vi "Begin.vi"(8 "error in":errorcluster) -> (0 "error out":errorcluster)   [LabVIEW 2020]
doc: "Called before other user functions, this VI is expected to open initial I/O refnums, load in file data, and do all program initialization. Notice that the <B>error out</B> terminal is simply used for data flow. Wiring it to other structures or subVIs ensures that this VI runs first."
uses:
  <vilib>/Rock Robotics/WPI/DriverStation/WPI_DriverStationRobotMode2.ctl
  Robot Global Data.vi
  <vilib>/Rock Robotics/Network Tables/NT Write String Array.vi
panel:
  in  "Drive Can Id":T1={"Front Left Drive CAN"=2, "Front Right Drive CAN"=3, "Back Left Drive CAN"=8, "Back Right Drive CAN"=5}
  in  "Steer Can Id":T2={"Front Left  Steer CAN"=6, "Front Right Steer CAN"=7, "Back Left Steer CAN"=9, "Back Right Steer CAN"=4}
  in  "Wheel Base Width":dbl=24.0
  in  "Wheel Base Length":dbl=24.0
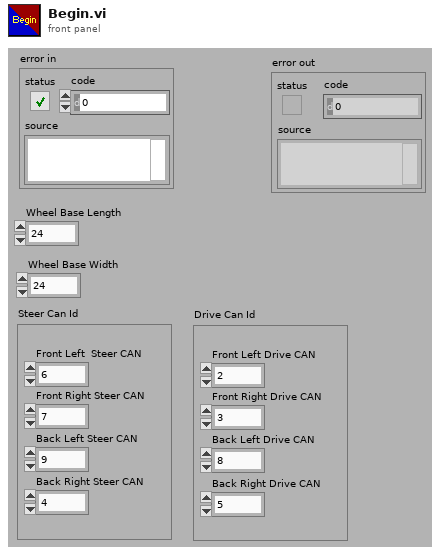
[diagram p1: front panel]
types:
  T1 = cluster{"Front Left Drive CAN":u8, "Front Right Drive CAN":u8, "Back Left Drive CAN":u8, "Back Right Drive CAN":u8}
  T2 = cluster{"Front Left  Steer CAN":u8, "Front Right Steer CAN":u8, "Back Left Steer CAN":u8, "Back Right Steer CAN":u8}
  T3 = typedef "WPI_DriverStationRobotMode2.ctl" = enum16{"Autonomous Disabled", "Autonomous Enabled", "Teleop Disabled", "Teleop Enabled", "Disconnected", "Finish", "Test Disabled", "Test Enabled", "Emergency Stopped"}
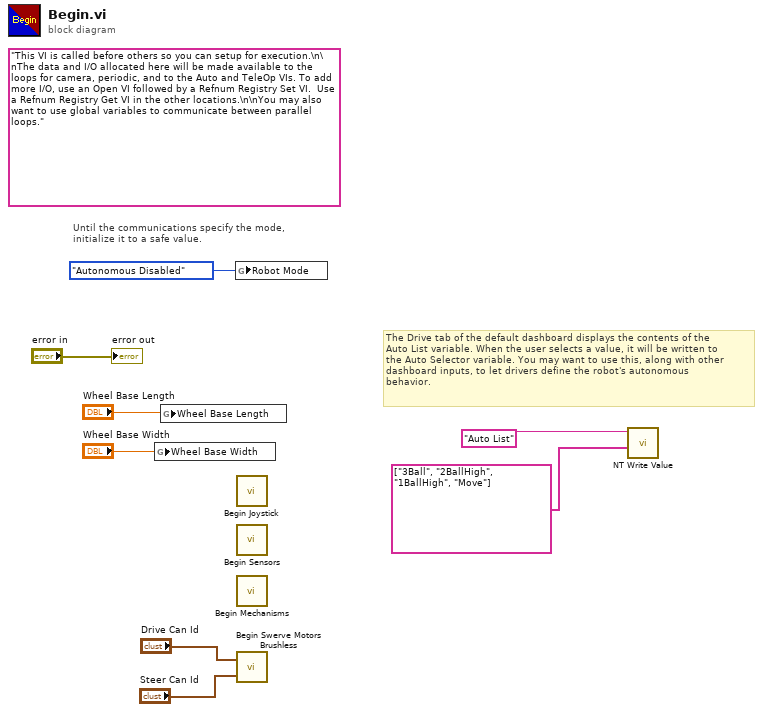
[diagram p0: block diagram]
diagram:
  (unwired) "This VI is called before others so you can setup for execution.\n\nThe data and I/O allocated here will be made available to the loops for camera, periodic, and to the Auto and TeleOp VIs. To add more I/O, use an Open VI followed by a Refnum Registry Set VI.  Use a Refnum Registry Get VI in the other locations.\n\nYou may also want to use global variables to communicate between parallel loops."
  # "The Drive tab of the default dashboard displays the contents of the\nAuto List variable. When the user selects a value, it will be written to\nthe Auto Selector variable. You may want to use this, along with other\ndashboard inputs, to let drivers define the robot's autonomous\nbehavior."
  # "Until the communications specify the mode,\ninitialize it to a safe value."
  n1 = global write "Robot Global Data.vi" "Wheel Base Width"("Wheel Base Width") -> ()
  n2 = global write "Robot Global Data.vi" "Wheel Base Length"("Wheel Base Length") -> ()
  n3 = global write "Robot Global Data.vi" "Robot Mode"(WPI_DriverStationRobotMode2."Autonomous Disabled" ("Robot Mode")) -> ()
  n4 = call "Begin Joystick.vi"() -> ()  [unwired: 12 in]
  n5 = call "Begin Sensors.vi"() -> ()  [unwired: 12 in]
  n6 = call "Begin Mechanisms.vi"() -> ()  [unwired: 12 in]
  n7 = call "Begin Swerve Motors Brushless.vi"("Steer Can Id"="Steer Can Id", "Drive Can Id"="Drive Can Id") -> ()  [unwired: 2 in]
  n8 = call-poly <vilib>:"NT Write Value.vi"("String Array"=string[] ["3Ball", "2BallHigh", "1BallHigh", "Move"], "Name"="Auto List") -> ()  [unwired: 9 in, 1 out]
  "error out" <- "error in"
